vi "Delete Target Module.vi"(0 "BroadcastRegistry In":T1, 7 "TargetCSM":string) -> (4 "BroadcastRegistry Out":T1)   [LabVIEW 2017, in "Communicable State Machine.lvlib"]
doc: "### Delete Target Module.vi\n\n-- <b>Controls</b> --\n- <b>BroadcastRegistry in</b>:\n- <b>Source</b>:\n\n-- <b>Indicators</b> --\n- <b>BroadcastRegistry out</b>:"
uses:
  Communicable State Machine.lvlib
  BroadcastRegistry.ctl
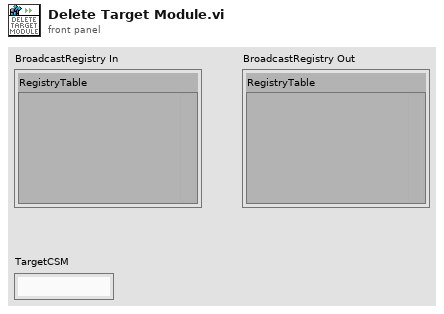
[diagram p1: front panel]
types:
  T1 = typedef "Communicable State Machine.lvlib/BroadcastRegistry.ctl" = cluster{"RegistryTable":variant}
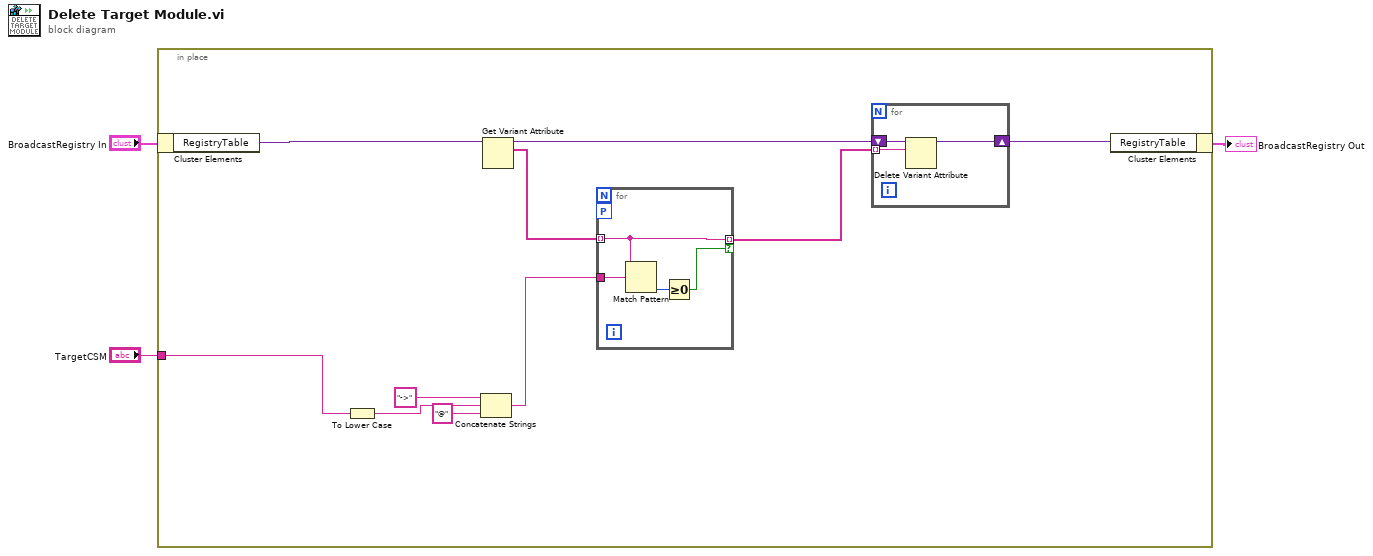
[diagram p0: block diagram]
diagram:
  n1 = in-place {
    in-place-border: "TargetCSM" -> [w4]
    n2 = in-place-cluster #1("BroadcastRegistry In") -> ("RegistryTable"=w13:variant)
    n3 = To Lower Case(string=w4) -> (all lower case string=w10:string)
    n4 = Concatenate Strings("->" ("string"), w10, "@" ("string")) -> (w6:string)
    n5 = Get Variant Attribute(Variant=w13) -> (duplicate Variant=w9:variant, names=w8:string[])  [unwired: 3 in, 2 out]
    n6 = for {
      tunnel: w8 -> [w20] mode=indexing
      tunnel: [w20] -> w7 mode=indexing if=w17
      tunnel: w6 -> [w19]
      workers-P: _ -> [_]
      n7 = Match Pattern(string=w20, regular expression=w19) -> (offset past match=w18:i32)  [unwired: 1 in, 3 out]
      n8 = Greater Or Equal To 0?(x=w18) -> (x >= 0?=w17:bool)
    }
    n9 = for {
      tunnel: w7 -> [w14] mode=indexing
      shift-right: [w16] -> w5
      shift-left: w9 -> [w15]
      n10 = Delete Variant Attribute(6:w14, 7:w15) -> (3:w16:variant)  [unwired: 1 in, 2 out]
    }
    n11 = in-place-cluster #1("RegistryTable"=w5) -> (→"BroadcastRegistry Out":T1)
  }
